vi "Set Poll Parameters.vi"(8 "error in (no error)":errorcluster, 10 "Poll Frequency (ms)":i32=-1, 11 "Actor Monitor in":refnum<class "Actor Monitor.lvclass">) -> (0 "error out":errorcluster, 3 "Actor Monitor out":refnum<class "Actor Monitor.lvclass">)   [LabVIEW 2018, in "Monitored Actor.lvlib" / "Actor Monitor.lvclass"]
doc: "Sets up a new periodic poller\n\nCopyright: MGI\nAuthored by: Derek Trepanier"
uses:
  Actor Monitor.lvclass
  C:/Program Files (x86)/National Instruments/LabVIEW 2018/vi.lib/ActorFramework/Actor/Actor.lvclass
  <vilib>/ActorFramework/Actor/Actor.lvclass/Actor.ctl
  <vilib>/ActorFramework/Message Enqueuer/Message Enqueuer.lvclass/Message Enqueuer.ctl
  Actor Monitor.lvclass/Actor Monitor.ctl
  Actor Monitor Messages/Ping Actors Msg/Ping Actors Msg.lvclass
  C:/Program Files (x86)/National Instruments/LabVIEW 2018/vi.lib/ActorFramework/Message/Message.lvclass
  <vilib>/ActorFramework/Message Enqueuer/Init from Existing Queue.vi
  <vilib>/ActorFramework/Message Enqueuer/Message Enqueuer.lvclass
  <vilib>/ActorFramework/Actor/Actor.lvclass
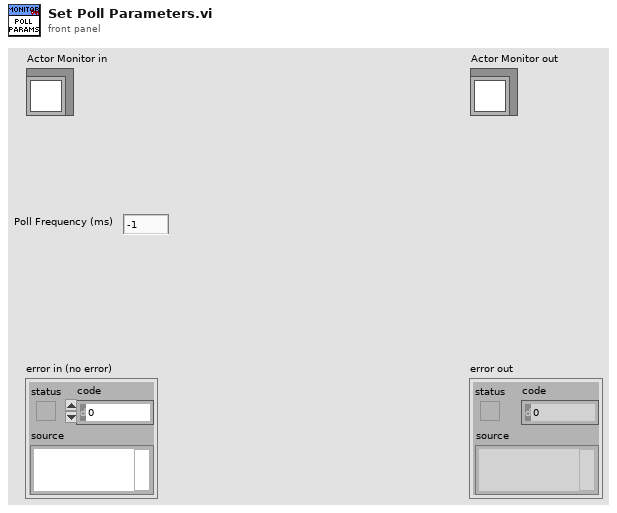
[diagram p1: front panel]
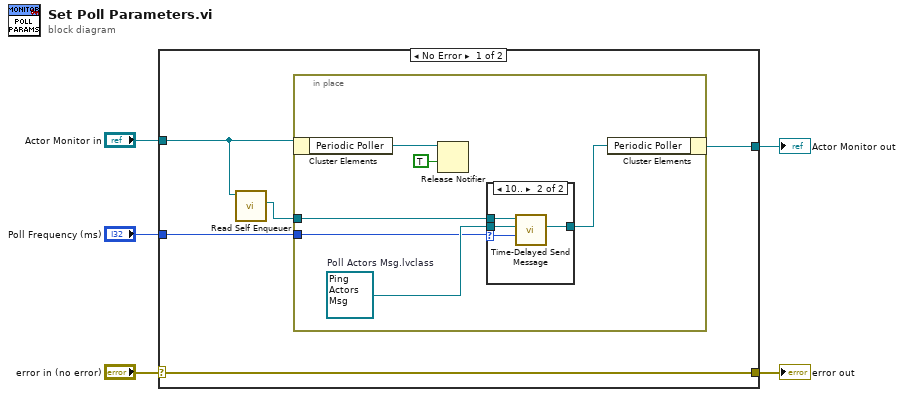
[diagram p0: block diagram]
diagram:
  n1 = case shown="No Error" "error in (no error)" {
    selector: "error in (no error)" -> [w10 w22]
    tunnel: [w10 w22] -> w4
    tunnel: [w9 w21] -> w2
    tunnel: "Actor Monitor in" -> [w7 w21]
    tunnel: "Poll Frequency (ms)" -> [w8 _]
    frame No Error {
      n2 = call <vilib>:"Read Self Enqueuer.vi"("Actor"=w7) -> ("Self Enqueuer"=w6:refnum<class "Message Enqueuer.lvclass">)  [unwired: 10 in]
      n3 = in-place {
        in-place-border: w8 -> [w11]
        in-place-border: w6 -> [w14]
        w13 = refnum<class "Ping Actors Msg.lvclass"> refnum  # Poll Actors Msg.lvclass
        n4 = in-place-cluster #1(w7) -> ("Periodic Poller"=w16:refnum<notifier>)
        n5 = Release Notifier(notifier=w16, force destroy? (F)=TRUE) -> ()  [unwired: 1 in, 3 out]
        n6 = case shown="10.." w11 {
          selector: w11 -> [_ w17]
          tunnel: w14 -> [_ w20]
          tunnel: w13 -> [_ w19]
          tunnel: [_ w18] -> w12
          frame Default {
          }
          frame 10.. {
            n7 = call <vilib>:"Time-Delayed Send Message.vi"("Milliseconds To Wait"=w17, "Message"=w19, "Message Enqueuer"=w20) -> ("Delivery Notifier"=w18:refnum<notifier>)  [unwired: 7 in, 1 out]
          }
        }
        n8 = in-place-cluster #1("Periodic Poller"=w12) -> (w9:refnum<class "Actor Monitor.lvclass">)
      }
    }
    frame Error {
    }
  }
  "error out" <- w4
  "Actor Monitor out" <- w2
